vi "LINX - Analog Read - TCP Interface.vi"() -> ()   [LabVIEW 2011, in "LVH-LINX.lvlib"]
doc: "Read one or more analog values from a LINX device using the LINX TCP interface."
uses:
  vi.lib/LabVIEW Hacker/LINX/LVH-LINX.lvlib
  vi.lib/LabVIEW Hacker/LINX/Private/Device/Type Defs/TCP Config.ctl
  vi.lib/LabVIEW Hacker/LINX/Private/Type Defs/Interface.ctl
  vi.lib/LabVIEW Hacker/LINX/Private/Device/Device.lvlib
panel:
  in  "TCP Configuration":T1
  in  "AI Channel(s)":u8[](array[numeric])=[0, 1, 2]
  out "Loop Rate (Hz)":u32
  in  "Stop Button":bool
  out "Analog Data":T2(graph)
  # "Circuit Schematic"
  # "LINX Device Settings"
  # "Analog Values"
  # "Analog Read Example (TCP Interface)\n\nThis example demonstrates how to read analog input values from a LINX device connected to the host computer via Serial / USB.\n\nInstructions\n1. Enter the IP Addres and Port associated with the LINX Device.\n2. Select the Analog Channel(s) to read.\n3. Click the Run Arrow."
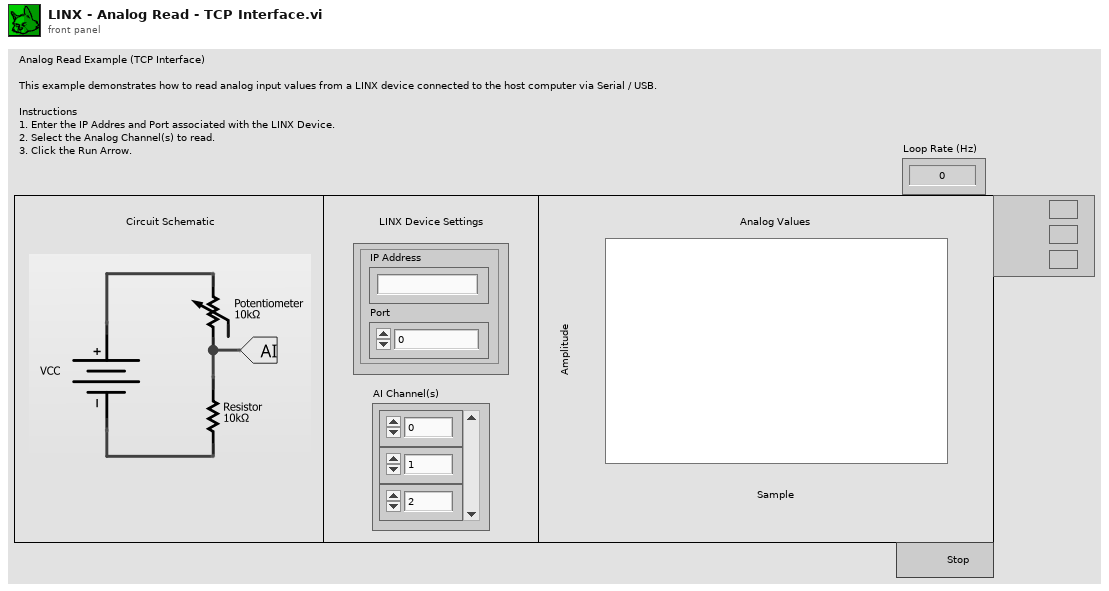
[diagram p1: front panel]
types:
  T1 = typedef "LVH-LINX.lvlib/Device.lvlib/TCP Config.ctl" = cluster{"IP Address":string, "Port":u16}
  T2 = cluster{"Voltages[0]":dbl, "Voltages[1]":dbl, "Voltages[2]":dbl, "Voltages[3]":dbl, "Voltages[4]":dbl, "Voltages[5]":dbl, "Voltages[6]":dbl, "Voltages[7]":dbl, "Voltages[8]":dbl}
  T3 = typedef "LVH-LINX.lvlib/Interface.ctl" = enum16{"Serial", "TCP"}
  T4 = typedef "LVH-LINX.lvlib/LINX Ref.ctl" = cluster{"Platform":T5, "Interface":T3, "LINX Device Config":T6}
  T5 = typedef "LVH-LINX.lvlib/Platform.ctl" = enum16{"LINX", "myRIO"}
  T6 = typedef "LVH-LINX.lvlib/Device.lvlib/LINX Device Config.ctl" = cluster{"Interface":T3, "COM Port":refnum<visa-resource-name>, "TCP Configuration":T1, "Device Family":T7, "Device ID":u8, "Device Name":string, "TCP Ref":refnum<k5>}
  T7 = typedef "LVH-LINX.lvlib/Device Family.ctl" = enum8{"National Instruments", "Digilent", "Arduino"}
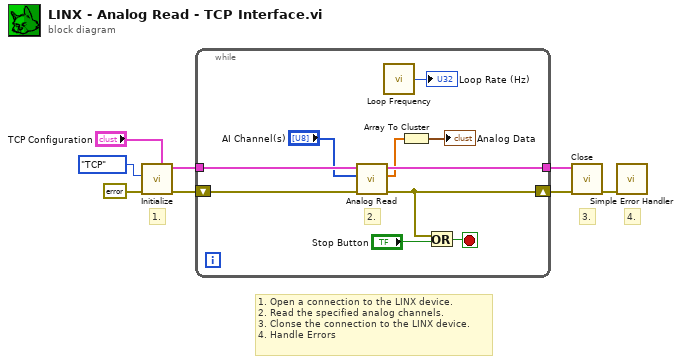
[diagram p0: block diagram]
diagram:
  # "1. Open a connection to the LINX device.\n2. Read the specified analog channels.\n3. Clonse the connection to the LINX device.\n4. Handle Errors"
  # "4."
  # "3."
  # "1."
  n1 = call "Initialize.vi"("TCP Configuration"="TCP Configuration", "Error In"=errorcluster {"status"=FALSE, "code"=0, "source"=""}, "Interface"=Interface."TCP") -> ("Error Out"=w7:errorcluster, "LINX Ref"=w8:T4)  [unwired: 6 in, 1 out]
  n2 = while {
    tunnel: w8 -> [w18]
    tunnel: [w16] -> w6
    shift-right: [w14] -> w5
    shift-left: w7 -> [w17]
    stop <- w15 stop-if-true
    # "2."
    n3 = call "Analog Read.vi"("Error In"=w17, "AI Channel(s)"="AI Channel(s)", "LINX Resource"=w18) -> ("Error Out"=w14:errorcluster, "Voltages"=w13:dbl[], "LINX Resource"=w16:T4)  [unwired: 5 in, 1 out]
    n4 = call "Loop Frequency.vi"() -> ("Loop Rate (Hz)"=→"Loop Rate (Hz)":u32)
    n5 = Array To Cluster(array=w13) -> (cluster=→"Analog Data":T2)
    n6 = Or(x=w14, y="Stop Button") -> (x .or. y?=w15:bool)
  }
  n7 = call "Close.vi"("Error In"=w5, "LINX Resource"=w6) -> ("Error Out"=w4:errorcluster)  [unwired: 8 in, 1 out]
  n8 = call <vilib>:"Simple Error Handler.vi"("error in (no error)"=w4) -> ()  [unwired: 4 in, 5 out]
